vi "Camera Capabilities.vi"() -> ()   [LabVIEW 2018]
uses:
  <userlib>/atmcd32d.llb/AndorCapabilities typedef.ctl
  CCDCamera/CCDCamera.lvclass
  <userlib>/atmcd32d.llb/HSSpeed_type typedef.ctl
panel:
  out "InternalShutter":i32
  out "Camera Capabilities":T1
  out "VSSpeed":dbl[](array[numeric])
  out "Conventional HSSpeed":dbl[](array[numeric])
  out "EM HSSpeed":dbl[](array[numeric])
  out "Pixel depth":i32
  out "# PreAmps":i32
  out "# AD Channel":i32
  # "Characterization of the Camera Capabilities"
  # "obs: a camera pode ter mais recursos que não são mostrados no Cluster."
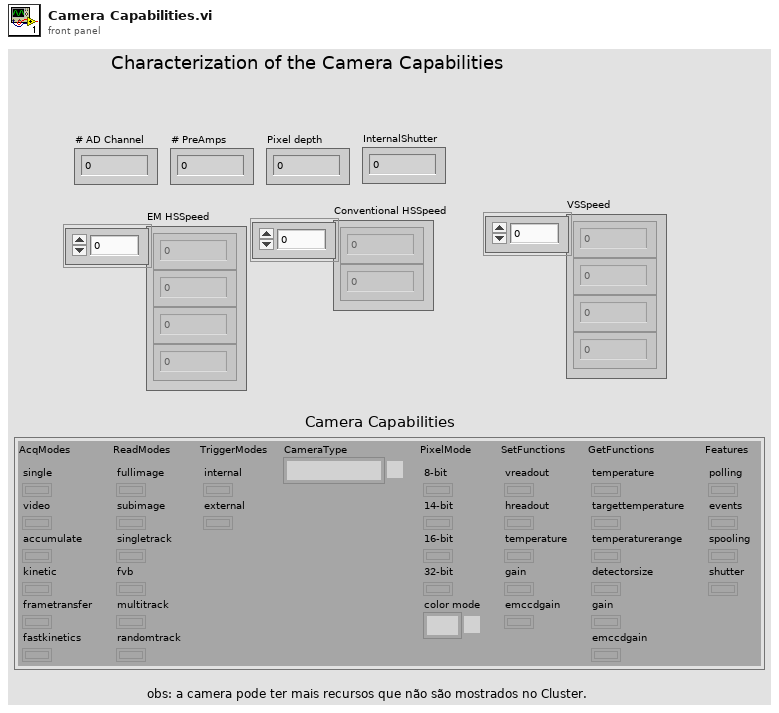
[diagram p1: front panel]
types:
  T1 = typedef "AndorCapabilities typedef.ctl" = cluster{"AcqModes":cluster{"single":bool, "video":bool, "accumulate":bool, "kinetic":bool, "frametransfer":bool, "fastkinetics":bool}, "ReadModes":cluster{"fullimage":bool, "subimage":bool, "singletrack":bool, "fvb":bool, "multitrack":bool, "randomtrack":bool}, "TriggerModes":cluster{"internal":bool, "external":bool}, "CameraType":enum32{"PDA", "iXon", "ICCD", "EMCCD", "CCD", "iStar", "third party camera", "iDus", "Newton", "Surcam", "USB ICCD", "Luca", "Reserved", "iKon", "InGaAs", "iVac", "Unprogrammed", "Clara", "USB iStar", "SimCam", "Neo", "iXon Ultra", "Volmos", "iVac Ultra"}, "PixelMode":cluster{"8-bit":bool, "14-bit":bool, "16-bit":bool, "32-bit":bool, "color mode":enum16{"Mono", "RGB", "CMY"}}, "SetFunctions":cluster{"vreadout":bool, "hreadout":bool, "temperature":bool, "gain":bool, "emccdgain":bool}, "GetFunctions":cluster{"temperature":bool, "targettemperature":bool, "temperaturerange":bool, "detectorsize":bool, "gain":bool, "emccdgain":bool}, "Features":cluster{"polling":bool, "events":bool, "spooling":bool, "shutter":bool}}
  T2 = typedef "HSSpeed_type typedef.ctl" = enum16{"EM Amp", "Conventional Amp"}
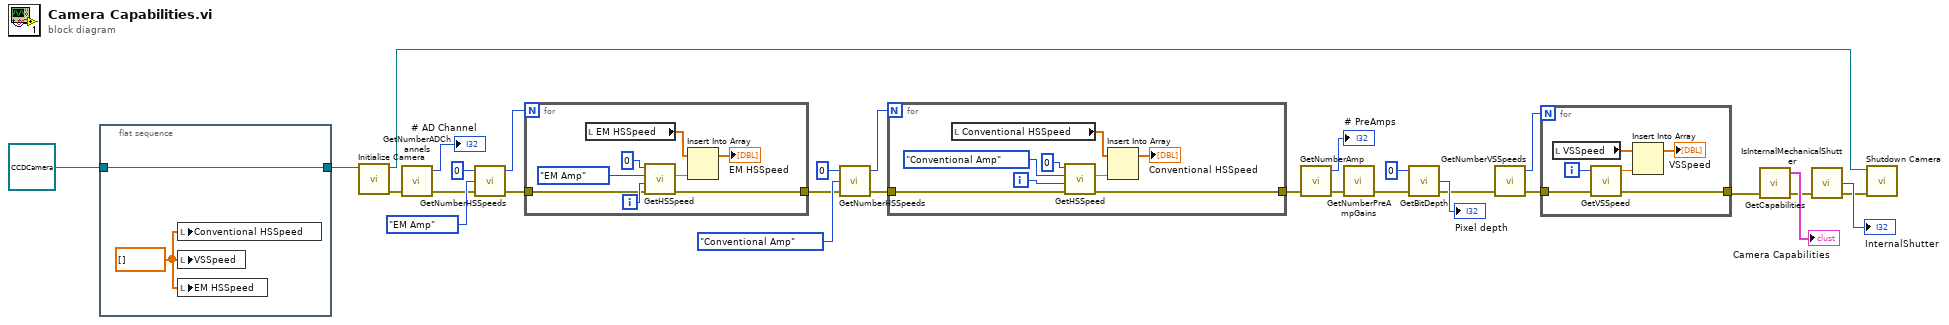
[diagram p0: block diagram]
diagram:
  n1 = flat-sequence {
    tunnel: refnum<class "CCDCamera.lvclass"> refnum ("CCDCamera in") -> [w30]
    tunnel: [w30] -> w6
    frame #0 {
      w31 = dbl[] []
      n2 = local write "Conventional HSSpeed"(w31) -> ()
      n3 = local write "VSSpeed"(w31) -> ()
      n4 = local write "EM HSSpeed"(w31) -> ()
    }
  }
  n5 = call "Initialize Camera.vi"("CCDCamera in"=w6) -> ("error out"=w28:errorcluster, "CCDCamera out"=w27:refnum<class "CCDCamera.lvclass">)  [unwired: 9 in]
  n6 = call <userlib>:"GetNumberADChannels.vi"("error in (no error)"=w28) -> ("error out"=w19:errorcluster, "number"=→"# AD Channel":i32)  [unwired: 2 in, 1 out]
  n7 = call <userlib>:"GetNumberHSSpeeds.vi"("error in (no error)"=w19, "type"=HSSpeed_type_typedef."EM Amp", "channel"=0) -> ("error out"=w16:errorcluster, "number"=w17:i32)  [unwired: 1 out]
  n8 = for {
    N: w17 -> [_]
    tunnel: w16 -> [w33]
    tunnel: [w32] -> w12
    i -> [w35]
    n9 = local read "EM HSSpeed"() -> (w39:dbl[])
    n10 = call <userlib>:"GetHSSpeed.vi"("error in (no error)"=w33, "index"=w35, "type"=HSSpeed_type_typedef."EM Amp", "channel"=0) -> ("error out"=w32:errorcluster, "speed"=w34:sgl)  [unwired: 1 in, 1 out]
    n11 = Insert Into Array(array=w39, new element=w34) -> (→"EM HSSpeed":dbl[])  [unwired: 1 in]
  }
  n12 = call <userlib>:"GetNumberHSSpeeds.vi"("error in (no error)"=w12, "type"=HSSpeed_type_typedef."Conventional Amp", "channel"=0) -> ("error out"=w11:errorcluster, "number"=w15:i32)  [unwired: 1 out]
  n13 = for {
    N: w15 -> [_]
    tunnel: w11 -> [w42]
    tunnel: [w41] -> w10
    i -> [w44]
    n14 = local read "Conventional HSSpeed"() -> (w47:dbl[])
    n15 = call <userlib>:"GetHSSpeed.vi"("error in (no error)"=w42, "index"=w44, "type"=HSSpeed_type_typedef."Conventional Amp", "channel"=0) -> ("error out"=w41:errorcluster, "speed"=w43:sgl)  [unwired: 1 in, 1 out]
    n16 = Insert Into Array(array=w47, new element=w43) -> (→"Conventional HSSpeed":dbl[])  [unwired: 1 in]
  }
  n17 = call <userlib>:"GetNumberAmp.vi"("error in (no error)"=w10) -> ("error out"=w26:errorcluster, "number"=→"# PreAmps":i32)  [unwired: 2 in, 1 out]
  n18 = call <userlib>:"GetNumberPreAmpGains.vi"("error in (no error)"=w26) -> ("error out"=w25:errorcluster)  [unwired: 2 in, 2 out]
  n19 = call <userlib>:"GetBitDepth.vi"("error in (no error)"=w25, "channel"=0) -> ("error out"=w18:errorcluster, "depth"=→"Pixel depth":i32)  [unwired: 1 in, 1 out]
  n20 = call <userlib>:"GetNumberVSSpeeds.vi"("error in (no error)"=w18) -> ("error out"=w9:errorcluster, "number"=w8:i32)  [unwired: 2 in, 1 out]
  n21 = for {
    N: w8 -> [_]
    tunnel: w9 -> [w49]
    tunnel: [w48] -> w5
    i -> [w52]
    n22 = local read "VSSpeed"() -> (w53:dbl[])
    n23 = call <userlib>:"GetVSSpeed.vi"("error in (no error)"=w49, "index"=w52) -> ("error out"=w48:errorcluster, "speed"=w50:sgl)  [unwired: 1 in, 1 out]
    n24 = Insert Into Array(array=w53, new element=w50) -> (→"VSSpeed":dbl[])  [unwired: 1 in]
  }
  n25 = call <userlib>:"GetCapabilities.vi"("error in (no error)"=w5) -> ("error out"=w3:errorcluster, "caps"=→"Camera Capabilities":T1)  [unwired: 2 in, 1 out]
  n26 = call <userlib>:"IsInternalMechanicalShutter.vi"("error in (no error)"=w3) -> ("error out"=w1:errorcluster, "InternalShutter"=→"InternalShutter":i32)  [unwired: 2 in, 1 out]
  n27 = call "Shutdown Camera.vi"("error in (no error)"=w1, "CCDCamera in"=w27) -> ()  [unwired: 8 in, 2 out]
